vi "GlobalPlotUpdateTime.vi"() -> ()   [LabVIEW 2013]
panel:
  in  "Prev Time":dbl
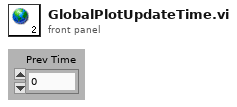
[diagram p1: front panel]
diagram:
